vi "lab 2.vi"(0 "String Input":string) -> (1 "Hz":dbl, 2 "V":dbl)   [LabVIEW 2014]
panel:
  out "Slope distance":dbl
  out "slope distance":string
  out "V":string
  out "Hz":string
  out "before substring":string
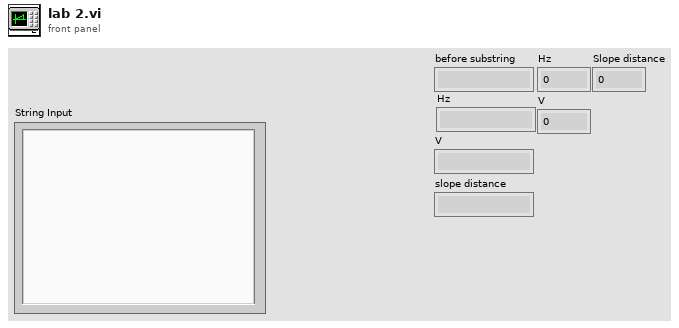
[diagram p1: front panel]
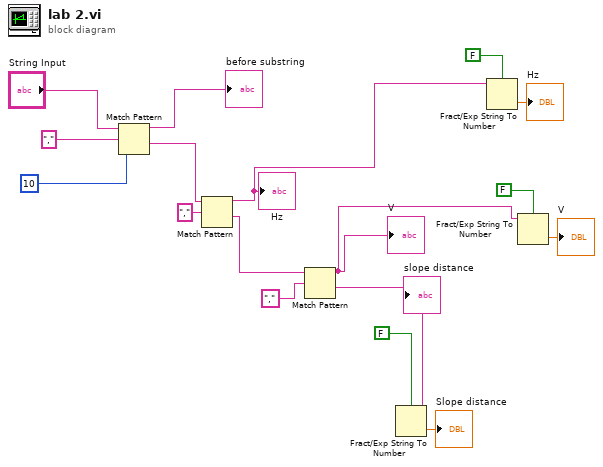
[diagram p0: block diagram]
diagram:
  n1 = Match Pattern(string="String Input", regular expression=",", offset (0)=10) -> (before substring=→"before substring":string, after substring=w1:string)  [unwired: 2 out]
  n2 = Match Pattern(string=w1, regular expression=",") -> (before substring=w10:string, after substring=w12:string)  [unwired: 1 in, 2 out]
  "Hz" <- w10
  n3 = Match Pattern(string=w12, regular expression=",") -> (before substring=w9:string, after substring=w8:string)  [unwired: 1 in, 2 out]
  "V" <- w9
  "slope distance" <- w8
  n4 = Fract/Exp String To Number(use system decimal point (T)=FALSE, string=w8) -> (number=→"Slope distance":dbl)  [unwired: 2 in, 1 out]
  n5 = Fract/Exp String To Number(use system decimal point (T)=FALSE, string=w10) -> (number=→"Hz":dbl)  [unwired: 2 in, 1 out]
  n6 = Fract/Exp String To Number(use system decimal point (T)=FALSE, string=w9) -> (number=→"V":dbl)  [unwired: 2 in, 1 out]
